vi "Interpolate (multiple).vi"(8 "error in (no error)":errorcluster, 10 "Configure":T1={"X Low"=0.05, "X High"=0.5, "X Step"=0.01, "Fake Point"=0.05} {"Fake Point" format="%#_6p"; "X Step" format="%#_6p"; "X High" format="%#_6p"; "X Low" format="%#_6p"}, 11 "XY-data":cluster{"X-array":dbl[], "Y-array":dbl[]}[](array[cluster]) {"Y-array" format="%.2p"; "X-array" format="%.2p"}) -> (0 "error out":errorcluster, 3 "Interpolated XY-data out":cluster{"X-array":dbl[], "Y-array":dbl[]}[](array[cluster]) {"Y-array" format="%.2p"; "X-array" format="%.2p"})   [LabVIEW 2019, in "xy_utilities.lvlib"]
doc: "Use this VI to interpolate data and add \"fake\" points outside of the given x array.\n\nThe <b>Configure</b> cluster is used to define:\n<b>X Low</b>: Starting x value for interpolation. May lie outside of the input x array range.\n<b>X High</b>: Ending x value for interpolation. May lie outside of the input x array range.\n<b>X Step</b>: Interpolation value.\n<b>Fake Point</b>: Value added to the y array for x values outside of the x array input range.\n\n\nWire data to the data input to determine the polymorphic instance to use or manually select the instance."
uses:
  xy_utilities.lvlib
  Typedefs/Interpolation Configuration--cluster.ctl
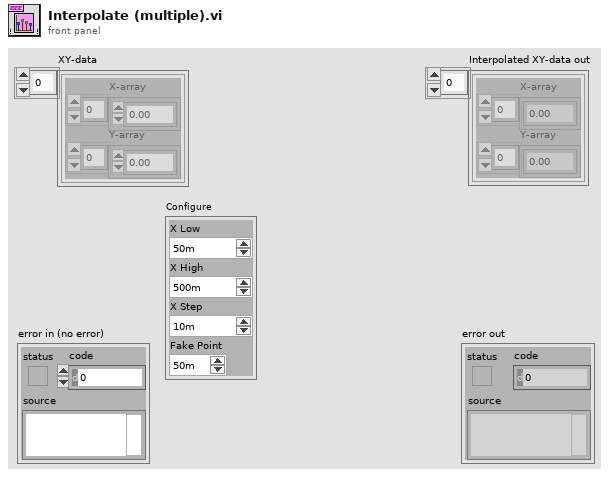
[diagram p1: front panel]
types:
  T1 = typedef "xy_utilities.lvlib/Interpolation Configuration--cluster.ctl" = cluster{"X Low":dbl, "X High":dbl, "X Step":dbl, "Fake Point":dbl}
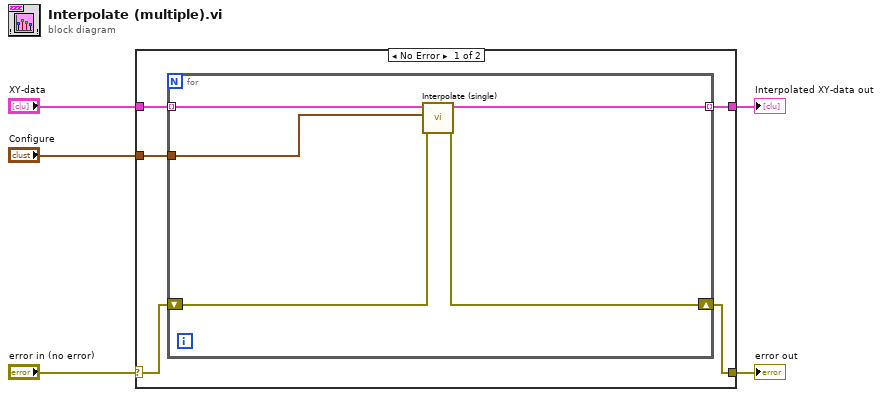
[diagram p0: block diagram]
diagram:
  n1 = case shown="No Error" "error in (no error)" {
    selector: "error in (no error)" -> [w8 w17]
    tunnel: [w7 w17] -> w4
    tunnel: "XY-data" -> [w10 w16]
    tunnel: [w9 w16] -> w2
    tunnel: "Configure" -> [w6 _]
    frame No Error {
      n2 = for {
        tunnel: w10 -> [w15] mode=indexing
        tunnel: [w14] -> w9 mode=indexing
        shift-right: [w11] -> w7
        shift-left: w8 -> [w12]
        tunnel: w6 -> [w13]
        n3 = call "Interpolate (single).vi"("error in (no error)"=w12, "Configure"=w13, "XY-data"=w15) -> ("error out"=w11:errorcluster, "Interpolated XY-data out"=w14:cluster{"X-array":dbl[], "Y-array":dbl[]})  [unwired: 7 in]
      }
    }
    frame Error {
    }
  }
  "error out" <- w4
  "Interpolated XY-data out" <- w2
